vi "update_event_data.vi"(8 "error in":errorcluster, 10 "JSON":string, 11 "event in":refnum<class "event.lvclass">) -> (0 "error out":errorcluster, 3 "event out":refnum<class "event.lvclass">)   [LabVIEW 2020, in "event.lvclass"]
uses:
  event.lvclass
  event.lvclass/event.ctl
  28bc5a72-9374-4728-b9ac-1639a12f899b.vi
  9860abd8-ae07-4152-ba21-12f5884466ca.vi
  7ff10bfd-9200-4696-87bf-282c67a758f1.vi
  <vilib>/JDP Science/JSONtext/Find Item.vi
  <vilib>/JDP Science/JSONtext/Next JSON Value.vi
  <vilib>/JDP Science/JSONtext/String Subset.vi
  <vilib>/JDP Science/JSONtext/Parsing/Advance past next JSON Value (inlined COPY).vi
  <vilib>/JDP Science/JSONtext/Parsing/Advance past whitespace.vi
  <vilib>/JDP Science/JSONtext/Parsing/Advance past String.vi
  <vilib>/JDP Science/JSONtext/Parsing/Advance past Number.vi
  <vilib>/JDP Science/JSONtext/Parsing/Advance past Line Ending.vi
  <vilib>/JDP Science/JSONtext/Parsing/Parse Full Path or Item Name.vi
  <vilib>/JDP Science/JSONtext/Parsing/Advance past Array.vi
  <vilib>/JDP Science/JSONtext/Parsing/Advance past Object.vi
  <vilib>/JDP Science/JSONtext/support/Error Cluster From Code.vi
  <vilib>/JDP Science/JSONtext/Offset/Find Item Locations by Path.vi
  <vilib>/JDP Science/JSONtext/JSON text to Variant.vi
  <vilib>/JDP Science/JSONtext/LVClass Serializer/JSONtext LVClass Serializer.lvclass
  <vilib>/JDP Science/JSONtext/JSONtext.lvlib
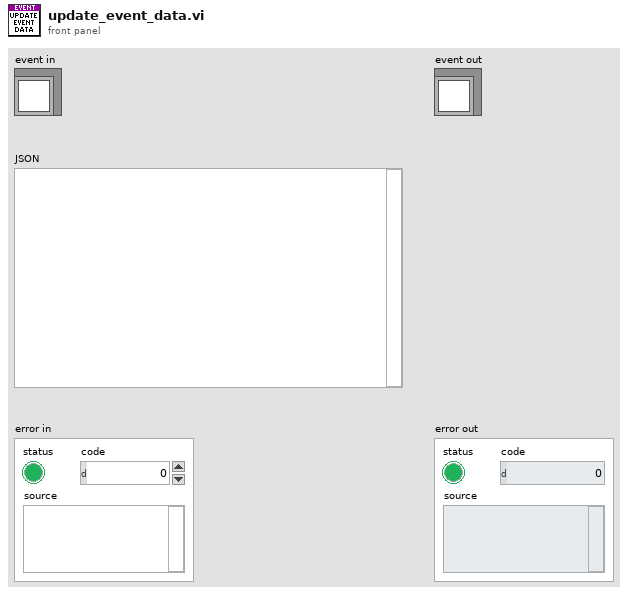
[diagram p1: front panel]
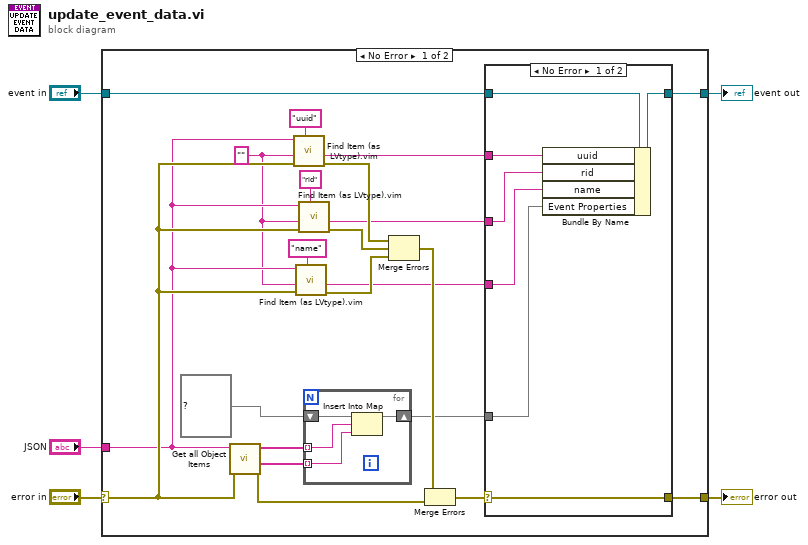
[diagram p0: block diagram]
diagram:
  n1 = case shown="No Error" "error in" {
    selector: "error in" -> [w27 w42]
    tunnel: "JSON" -> [w18 _]
    tunnel: "event in" -> [w15 w41]
    tunnel: [w14 w41] -> w5
    tunnel: [w12 w42] -> w1
    frame No Error {
      w9 = "" ("$Path or Item Name")
      n2 = call <vilib>:"Get all Object Items.vi"("error in (no error)"=w27, "JSON"=w18) -> ("error out"=w16:errorcluster, "<JSON>"=w25:string[], "Item Names"=w26:string[])  [unwired: 6 in, 1 out]
      n3 = call "Find Item (as LVtype).vim"("$Path or Item Name"="uuid", "error in (no error)"=w27, "Data Type and Default Value"=w9, "JSON"=w18) -> ("error out"=w21:errorcluster, "Data"=w8:string)  [unwired: 4 in, 2 out]
      n4 = call "Find Item (as LVtype).vim"("$Path or Item Name"="name", "error in (no error)"=w27, "Data Type and Default Value"=w9, "JSON"=w18) -> ("error out"=w19:errorcluster, "Data"=w6:string)  [unwired: 4 in, 2 out]
      n5 = call "Find Item (as LVtype).vim"("$Path or Item Name"="rid", "error in (no error)"=w27, "Data Type and Default Value"=w9, "JSON"=w18) -> ("error out"=w20:errorcluster, "Data"=w7:string)  [unwired: 4 in, 2 out]
      n6 = for {
        tunnel: w26 -> [w40] mode=indexing
        tunnel: w25 -> [w39] mode=indexing
        shift-right: [w37] -> w10
        shift-left: map{string, string} {} ("Event Properties") -> [w38]
        n7 = Insert Into Map(map in=w38, key=w40, value=w39) -> (map out=w37:map{string, string})  [unwired: 2 out]
      }
      n8 = Merge Errors(w21, w20, w19) -> (w17:errorcluster)
      n9 = Merge Errors(w17, w16) -> (w13:errorcluster)
      n10 = case shown="No Error" w13 {
        selector: w13 -> [w32 w35]
        tunnel: w15 -> [w34 w36]
        tunnel: [w33 w36] -> w14
        tunnel: [w32 w35] -> w12
        tunnel: w10 -> [w28 _]
        tunnel: w7 -> [w31 _]
        tunnel: w8 -> [w30 _]
        tunnel: w6 -> [w29 _]
        frame No Error {
          n11 = Bundle By Name(cluster=w34, "uuid"=w30, "rid"=w31, "name"=w29, "Event Properties"=w28) -> (w33:refnum<class "event.lvclass">)
        }
        frame Error {
        }
      }
    }
    frame Error {
    }
  }
  "event out" <- w5
  "error out" <- w1
